vi "Read LabJack Configuration.vi"(8 "error in (no error)":errorcluster, 11 "LabJack Driver in":refnum<class "LabJack Driver.lvclass">) -> (0 "error out":errorcluster, 2 "Configuration":T1={"Scale"=nan, "Offset"=0.0}, 3 "LabJack Driver out":refnum<class "LabJack Driver.lvclass">)   [LabVIEW 2021, in "LabJack Driver.lvclass"]
uses:
  LabJack Driver.lvclass
  C:/GitHub/NHMFL_Core/Libraries/Instruments/Instrument Driver/Instrument Driver.lvclass
  LabJack Configuration.ctl
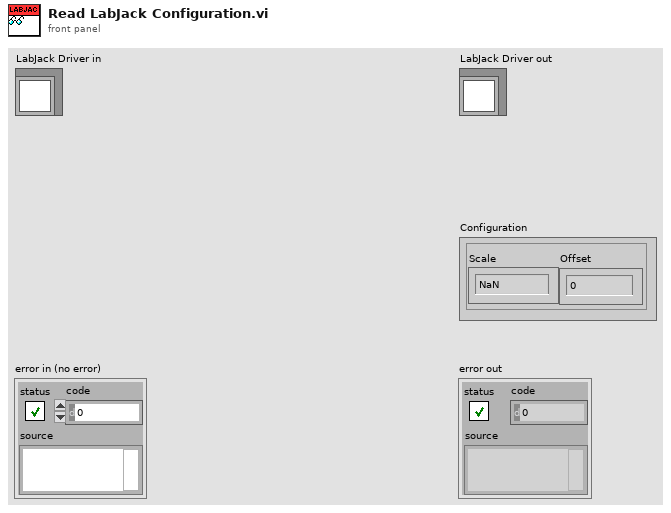
[diagram p1: front panel]
types:
  T1 = typedef "LabJack Configuration.ctl" = cluster{"Scale":dbl, "Offset":dbl}
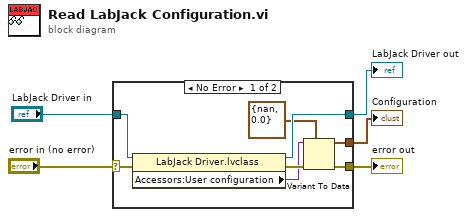
[diagram p0: block diagram]
diagram:
  n1 = case shown="No Error" "error in (no error)" {
    selector: "error in (no error)" -> [w13 w14]
    tunnel: [w9 w14] -> w4
    tunnel: [w12 w15] -> w2
    tunnel: "LabJack Driver in" -> [w11 w15]
    tunnel: [w6 _] -> w1
    frame No Error {
      n2 = property class="LabJack Driver.lvclass"(reference=w11, error in=w13) -> (reference out=w12:refnum<class "LabJack Driver.lvclass">, error out=w10:errorcluster, "Accessors:User configuration"=w7:variant)
      n3 = Variant To Data(error in=w10, type=T1 {"Scale"=nan, "Offset"=0.0} ("LabJack Configuration"), Variant=w7) -> (data=w6:T1, error out=w9:errorcluster)
    }
    frame Error {
    }
  }
  "error out" <- w4
  "LabJack Driver out" <- w2
  "Configuration" <- w1
